vi "ScopeCheck.vi"(2 "错误输入（无错误）":errorcluster) -> (0 "错误输出":errorcluster, 1 "通信正常？":bool)   [LabVIEW 2018]
uses:
  <instrlib>/Tektronix DPO MSO 2000 4000 Series/Tektronix DPO MSO 2000 4000 Series.lvlib
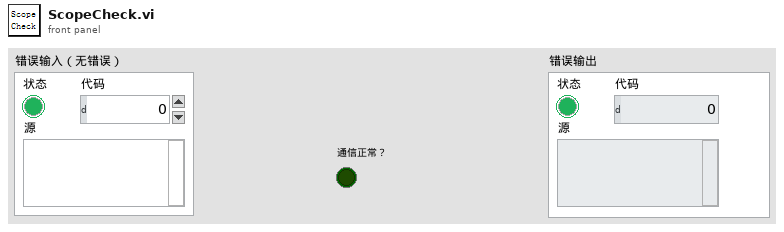
[diagram p1: front panel]
types:
  T1 = typedef "IMAQ Image.ctl" = refnum<image>
  T2 = cluster{"示波器":cluster{"Channel (0:Channel 1)":enum16{"Channel 1", "Channel 2", "Channel 3", "Channel 4"}, "电压范围":dbl, "触发电压":dbl, "时间范围":dbl, " 示波器VISA":refnum<visa-resource-name>, "时间范围 标签":u64, "电压范围 标签":u64, "触发电压 标签":u64}, "光谱仪":cluster{"SpecDataReference":refnum<queue>, "grating center":dbl, "Exposure Time (s)":dbl, "是否进行详细设置":bool, " 开始通信检查":bool, "通信成功？":bool, "波长":dbl}, " 近场相机":cluster{"曝光时间/100us":dbl, "模拟增益":i32, "控制套接字":i32, "IP 地址":string, " 采集套接字":i32, "  版本号":i32, "ImageData":T1, "  增益最大":i32, "  增益最小":i32, " 曝光最大":i32, " 曝光最小":i32, " 帧速":i32, " 同步切换":i32, "  曝光缩放":i32}, " 偏振仪":cluster{"电压范围":u64, "触发电压":u64, "时间范围":u64, "波长范围":enum16{"可见光 400-700nm", "近红外 700-1100nm"}, "可见光偏振测量仪VISA":refnum<visa-resource-name>, "近红外偏振测量仪VISA":refnum<visa-resource-name>}, " 功率计":cluster{"通道":enum16{"Channel 1", "Channel 2"}, "工作波长":u32, "单位":u64, "时间范围":u64, "IP地址":string, "端口":u32}, "能量计":cluster{"通道":enum16{"Channel 1", "Channel 2"}, "工作波长":u32, "单位":u64, "时间范围":u64, "IP地址":string, "端口":u32, "能量计量程":enum16{"200uJ", "20uJ", "2uJ", "200nJ"}}, "电机":cluster{"Channel (0:Channel 1)":enum16{"Channel 1", "Channel 2", "Channel 3", "Channel 4"}, "电压范围":u64, "触发电压":u64, "时间范围":u64}, " 远场相机":cluster{"曝光时间":i32, "模拟增益":i32, "控制套接字":i32, "IP 地址":string, " 采集套接字":i32, "  版本号":i32, "ImageData":T1, "  增益最大":i32, "  增益最小":i32, " 曝光最大":i32, " 曝光最小":i32, " 帧速":i32, " 同步切换":i32, "  曝光缩放":i32, "ImageData B":T1}}
  T3 = cluster{"Channel (0:Channel 1)":enum16{"Channel 1", "Channel 2", "Channel 3", "Channel 4"}, "电压范围":dbl, "触发电压":dbl, "时间范围":dbl, " 示波器VISA":refnum<visa-resource-name>, "时间范围 标签":u64, "电压范围 标签":u64, "触发电压 标签":u64}
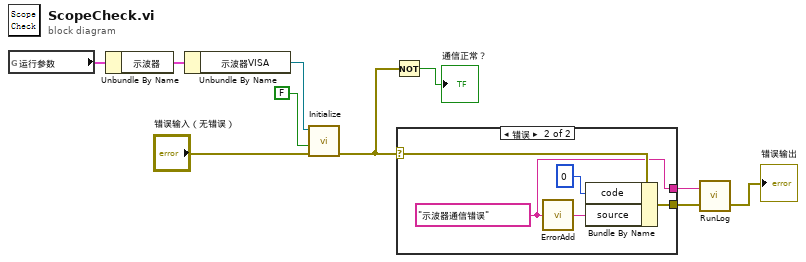
[diagram p0: block diagram]
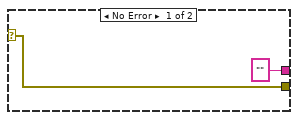
[diagram p2: hidden frame]
diagram:
  n1 = global read "参数.vi" "运行参数"() -> (w10:T2)
  n2 = Unbundle By Name(w10) -> ("示波器"=w9:T3)
  n3 = Unbundle By Name(w9) -> ("示波器VISA"=w8:refnum<visa-resource-name>)
  n4 = call <instrlib>:"Initialize.vi"("error in (no error)"="错误输入（无错误）", "Reset (True)"=FALSE, "VISA resource name"=w8) -> ("error out"=w2:errorcluster)  [unwired: 7 in, 1 out]
  n5 = Not(x=w2) -> (.not. x?=→"通信正常？":bool)
  n6 = case shown="错误" w2 {
    selector: w2 -> [w12 w15]
    tunnel: [w12 w14] -> w4
    tunnel: ["" ("source") w13] -> w5
    frame No Error {
    }
    frame Error {
      w13 = "示波器通信错误" ("source")
      n7 = call "ErrorAdd.vi"("source"=w13) -> ("Errorout Souce"=w16:string)
      n8 = Bundle By Name(cluster=w15, "code"=0, "source"=w16) -> (w14:errorcluster)
    }
  }
  n9 = call "RunLog.vi"("error in"=w4, "Message"=w5) -> ("error out"=→"错误输出":errorcluster)  [unwired: 1 in]
